vi "PH_ImageStatistician.Pack Dataset.vi"(0 "i ref in":refnum<vi>, 5 "error in":errorcluster) -> (14 "i ref out":refnum<vi>, 15 "Dataset Legend":string[](array[string]), 16 "Dataset chosen?":bool[](array[boolean]), 17 "Timebase":dbl[](array[numeric]), 18 "Dataset":dbl[][](array[numeric]), 19 "error out":errorcluster)   [LabVIEW 2014, in "PH_ImageStatistician.lvlib"]
doc: "This VI creates the dataset (Timebase, Data) out of the stored data."
uses:
  PH_ImageStatistician.lvlib
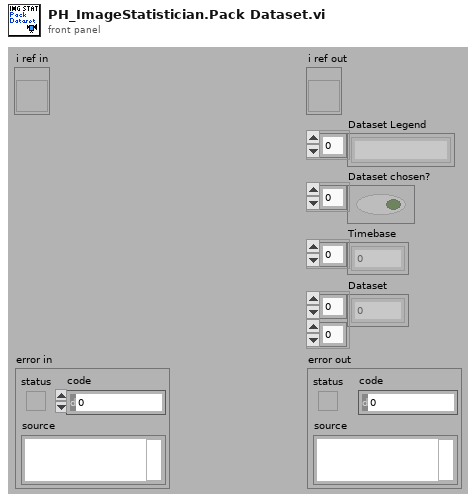
[diagram p1: front panel]
types:
  T1 = typedef "PH_ImageStatistician.lvlib/PH_ImageStatistician.i attribute.ctl" = cluster{"GUI Refs ":cluster{"Status":refnum<vi>, "Result Graph":refnum<vi>, "Mean Data 1":refnum<vi>, "Std Dev Data 1":refnum<vi>, "Mean Data 2":refnum<vi>, "Std Dev Data 2":refnum<vi>, "Mean Data 3":refnum<vi>, "Std Dev Data 3":refnum<vi>, "Dummy Mean":refnum<vi>, "Dummy Std Dev":refnum<vi>, "Export Data":refnum<vi>, "Data 1":refnum<vi>, "Data 2":refnum<vi>, "Data 3":refnum<vi>, "Stat or Trend":refnum<vi>, "Delete":refnum<vi>, "Operator":refnum<vi>, "Start":refnum<vi>}, "Operator":string, "Data":T2[], "Stat or Trend":bool, "Data 1":T3, "Data 2":T3, "Data 3":T3, "Start":bool, "Datasets strored":i32, "Dataarray Size":i32}
  T2 = typedef "PH_ImageStatistician.lvlib/PH_ImageStatistician.Statistician Data.ctl" = cluster{"Snapshot Time":dbl, "Maj FWHM":dbl, "Min FWHM":dbl, "Maj Fit Order":dbl, "Min Fit Order":dbl, "99% Diam Maj Trace":dbl, "99% Diam Min Trace":dbl, "Theta":dbl, "Delta":dbl, "Maj Diam":dbl, "Min Diam":dbl, "Azimuth Angle":dbl, "Azi Angle rel to major?":dbl, "Ellipticity":dbl, "CoG - X":dbl, "CoG - Y":dbl, "Energy":dbl, "Energy Cal - no mJ":dbl, "Lin Cal - no mm or mrad":dbl, "Lin Cal Factor":dbl}
  T3 = typedef "PH_ImageStatistician.lvlib/PH_ImageStatistician.select Data.ctl" = u16
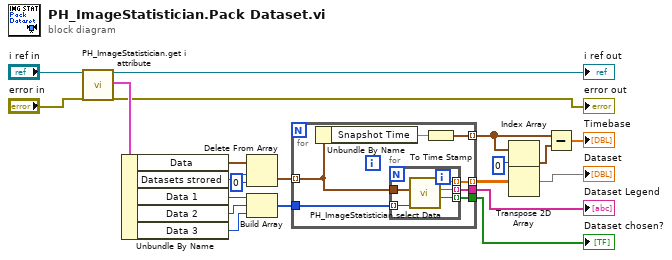
[diagram p0: block diagram]
diagram:
  n1 = call "PH_ImageStatistician.get i attribute.vi"("i ref in"="i ref in", "error in (no error)"="error in") -> ("i ref out"=→"i ref out":refnum<vi>, "i attribute"=w18:T1, "error out"=→"error out":errorcluster)  [unwired: 15 in]
  n2 = Unbundle By Name(w18) -> ("Data"=w4:T2[], "Datasets strored"=w3:i32, "Data 1"=w19:T3, "Data 2"=w20:T3, "Data 3"=w21:T3)
  n3 = Delete From Array(array=w4, length=w3, index=0) -> (deleted portion=w2:T2[])  [unwired: 1 out]
  n4 = Build Array(w19, w20, w21) -> (w7:T3[])
  n5 = for {
    tunnel: w2 -> [w28] mode=indexing
    tunnel: [w22] -> w8 mode=indexing
    tunnel: [w27] -> w10
    tunnel: [w26] -> w13
    tunnel: [w25] -> w9 mode=indexing
    tunnel: w7 -> [w24]
    n6 = Unbundle By Name(w28) -> ("Snapshot Time"=w23:dbl)
    n7 = for {
      tunnel: w28 -> [w30]
      tunnel: [w33] -> w27 mode=indexing
      tunnel: [w32] -> w26 mode=indexing
      tunnel: [w31] -> w25 mode=indexing
      tunnel: w24 -> [w29] mode=indexing
      n8 = call "PH_ImageStatistician.select Data.vi"("Data Selector"=w29, "Statistician Data"=w30) -> ("Data chosen?"=w32:bool, "Data Legend"=w33:string, "Data"=w31:dbl)  [unwired: 5 in]
    }
    n9 = To Time Stamp(1:w23) -> (0:w22:timestamp)
  }
  "Dataset chosen?" <- w13
  "Dataset Legend" <- w10
  n10 = Index Array(array=w8, index=0) -> (element=w5:timestamp)
  n11 = Transpose 2D Array(2D array=w9) -> (transposed array=→"Dataset":dbl[][])
  n12 = Subtract(x=w8, y=w5) -> (x-y=→"Timebase":dbl[])
